vi "PR4000 cfg get valve.vi"(8 "error in (no error)":errorcluster, 10 "Channel parsed command info":T1, 11 "MKS4000b in":refnum<class "ISSI_Iris.lvclass">) -> (0 "error out":errorcluster, 2 "new commands":string, 3 "MKS4000b out":refnum<class "ISSI_Iris.lvclass">)   [LabVIEW 2020]
uses:
  shared/CompressAndUpdate(Poly)/CompressAndUpdate(Enum).vi
  ISSI_Iris.lvclass
  C:/GEECS/Developers Version/source/Device Drivers/BaseDriver/BaseDriver.lvclass
  C:/GEECS/Developers Version/source/Device Drivers/ISSI_Iris/ISSI_Iris.lvclass
  Shared/Device Driver/channel parsed cmd cluster.ctl
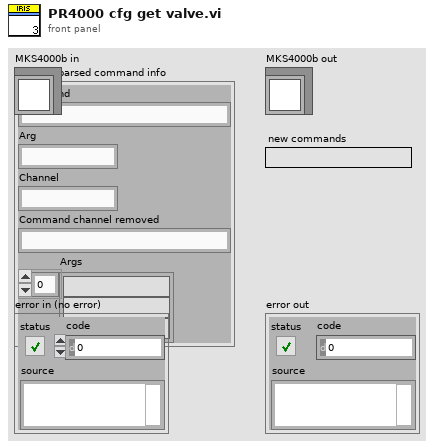
[diagram p1: front panel]
types:
  T1 = typedef "channel parsed cmd cluster.ctl" = cluster{"Command":string, "Arg":string, "Channel":string, "Command channel removed":string, "Args":string[]}
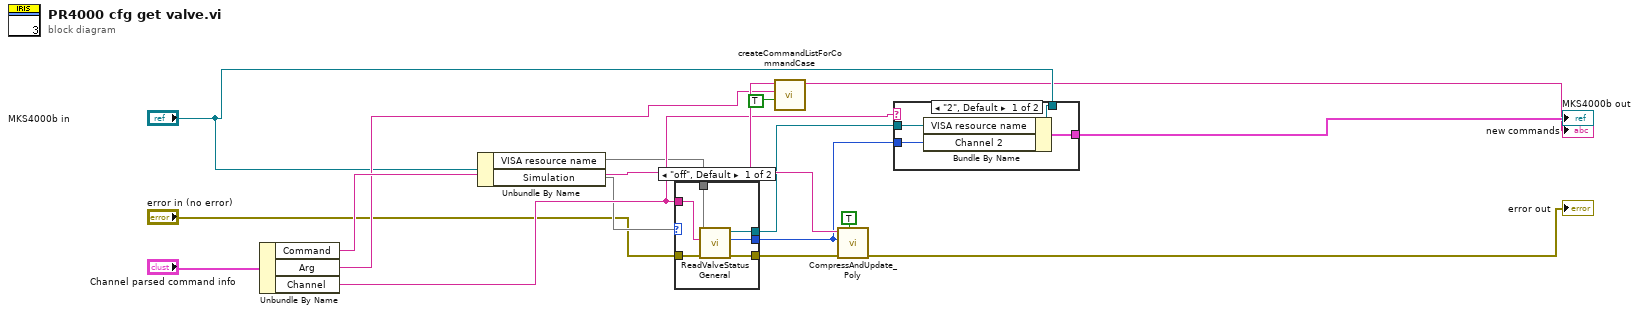
[diagram p0: block diagram]
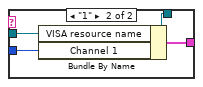
[diagram p2: hidden frame]
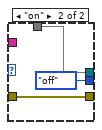
[diagram p3: hidden frame]
diagram:
  n1 = Unbundle By Name("Channel parsed command info") -> ("Command"=w16:string, "Arg"=w15:string, "Channel"=w14:string)
  n2 = Unbundle By Name("MKS4000b in") -> ("VISA resource name"=w4, "Simulation"=w7)
  n3 = case shown="\"off\", Default" w7 {
    tunnel: "error in (no error)" -> [w22 w23]
    tunnel: [w21 w23] -> w10
    tunnel: w14 -> [w20 _]
    tunnel: w4 -> [w19 w24]
    tunnel: [w18 w24] -> w11
    tunnel: [w17 enum16{"off", "on"}."off" ("Settings.Save")] -> w12
    frame "off", Default {
      n4 = call "ReadValveStatusGeneral.vi"("error in (no error)"=w22, "channel no in"=w20, "Comport PR4000"=w19) -> ("error out"=w21:errorcluster, "Settings.Save"=w17:enum16{"off", "on"}, "VISA resource name out"=w18:refnum<visa-resource-name>)  [unwired: 6 in]
    }
    frame "on" {
    }
  }
  n5 = call "createCommandListForCommandCase.vi"("immediate Check (only once)"=TRUE, "setvalue"=w15, "command"=w16) -> ("new commands"=→"new commands":string)  [unwired: 8 in]
  n6 = call-poly "CompressAndUpdate_Poly.vi"("force CVT update (false)"=TRUE ("force CVT update"), "error in"=w10, "enum variant"=w12, "command or variable name"=w16) -> ("error out"=→"error out":errorcluster)  [unwired: 7 in]
  n7 = case shown="\"2\", Default" w14 {
    tunnel: "MKS4000b in" -> [w29 w33]
    tunnel: [w28 w32] -> w6
    tunnel: w11 -> [w27 w31]
    tunnel: w12 -> [w26 w30]
    frame "2", Default {
      n8 = Bundle By Name(cluster=w29, "VISA resource name"=w27, "Channel 2"=w26) -> (w28:cluster{})
    }
    frame "1" {
      n9 = Bundle By Name(cluster=w33, "VISA resource name"=w31, "Channel 1"=w30) -> (w32:cluster{})
    }
  }
  "MKS4000b out" <- w6
